vi "global.vi"() -> ()   [LabVIEW 2024]
panel:
  out "Global Sample Rate":dbl
  out "Global System Status":enum16{"Automatic", "Manual", "Maintenance"}(ring)
  out "Global Heater Status":T1(ring)
  out "Global Current temperature reading":dbl(slide) scale=0.0..150.0
  out "Global Heater ON/OFF":bool
  out "Global Power ON/OFF":bool
  out "Global Historical Temperature Reading":dbl(graph)
  out "Global Temperature setpoint control Low":dbl
  out "Global Temperature setpoint control High":dbl
  out "Global Min Temperature Reading":dbl
  out "Global Max Temperature Reading":dbl
  out "Global Average Temperature (Last 5)":dbl
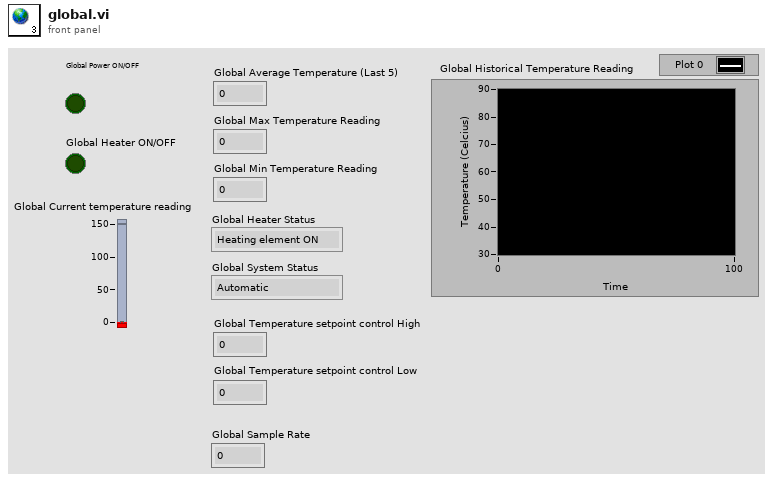
[diagram p1: front panel]
types:
  T1 = enum16{"Heating element ON", "Heating element OFF"}
diagram:
